vi "Test 5.vi"() -> ()   [LabVIEW 2015, in "Drona basic.lvlib"]
uses:
  Drona basic.lvlib
panel:
  in  "Numeric":dbl
  in  "Boolean":bool
  in  "Cluster":cluster{"Numeric":dbl, "Boolean":bool}
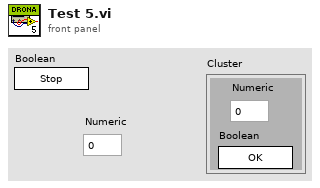
[diagram p1: front panel]
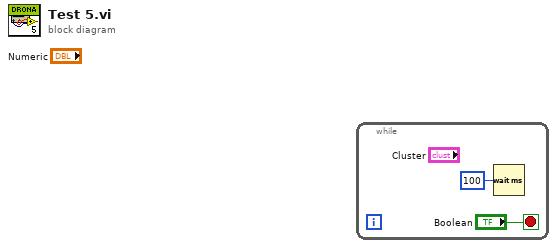
[diagram p0: block diagram]
diagram:
  n1 = while {
    stop <- "Boolean" stop-if-true
    n2 = Wait (ms)(milliseconds to wait=u32 100) -> ()  [unwired: 1 out]
  }
